vi "CB Discrete LQR.vi"(9 "R":T1, 10 "Q":T1, 11 "State Space Model":T2) -> (1 "X (ricatti solution)":T1, 3 "K (gain matrix)":T1)   [LabVIEW 2020]
uses:
  State-Space/CB State Space.ctl
  <vilib>/Analysis/Matrix/Datatypes/RealMatrix.ctl
  <vilib>/Analysis/7linalg.llb/Real Transpose Matrix.vi
  <vilib>/Analysis/baseanly.llb/Real A x B.vi
  <vilib>/Analysis/Matrix/Numeric/Add/Add - RM,RM.vi
  <vilib>/Analysis/7linalg.llb/Solve Linear Equations (multiple right hand).vi
  <vilib>/Analysis/NI_AALPro.lvlib
  <vilib>/Analysis/NI_AALBase.lvlib
  <vilib>/Analysis/Matrix/NI_Matrix.lvlib
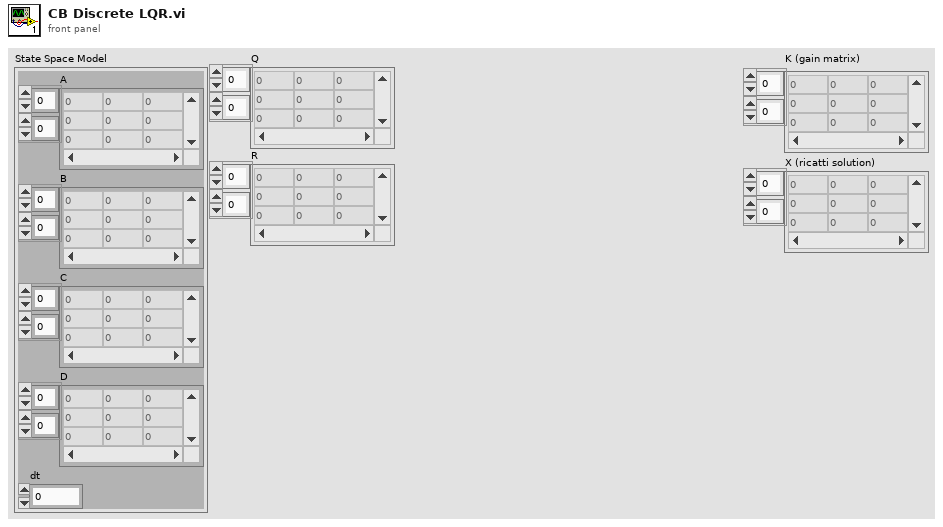
[diagram p1: front panel]
types:
  T1 = typedef "NI_Matrix.lvlib/RealMatrix.ctl" = dbl[][]
  T2 = typedef "CB State Space.ctl" = cluster{"A":T1, "B":T1, "C":T1, "D":T1, "dt":dbl}
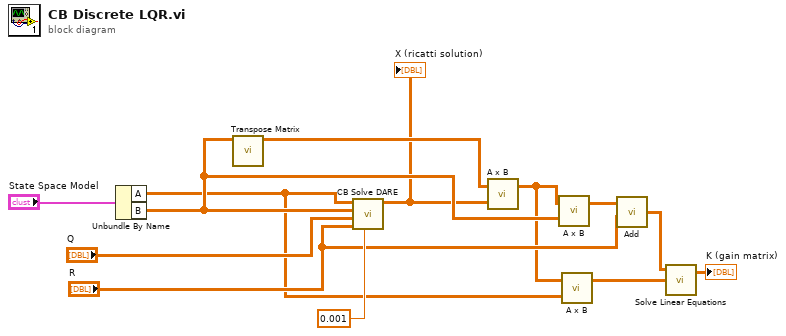
[diagram p0: block diagram]
diagram:
  n1 = Unbundle By Name("State Space Model") -> ("A"=w5:T1, "B"=w9:T1)
  n2 = call-poly <vilib>:"Transpose Matrix.vi"("Input Matrix"=w9) -> ("Matrix Transpose"=w10:T1)  [unwired: 9 in, 1 out]
  n3 = call "CB Solve DARE.vi"("epsilon"=0.001, "R"="R", "Q"="Q", "B"=w9, "A"=w5) -> ("X"=w1:T1)  [unwired: 6 in]
  "X (ricatti solution)" <- w1
  n4 = call-poly <vilib>:"A x B.vi"("B"=w1, "A"=w10) -> ("A x B"=w6:T1)  [unwired: 1 out]
  n5 = call-poly <vilib>:"A x B.vi"("B"=w9, "A"=w6) -> ("A x B"=w8:T1)  [unwired: 1 out]
  n6 = call-poly <vilib>:"A x B.vi"("B"=w5, "A"=w6) -> ("A x B"=w4:T1)  [unwired: 1 out]
  n7 = call-poly <vilib>:"Add.vi"("Real Matrix B"="R", "Real Matrix A"=w8) -> ("A + B"=w3:T1)
  n8 = call-poly <vilib>:"Solve Linear Equations.vi"("Known Matrix"=w4, "Input Matrix"=w3) -> ("Solution Matrix"=→"K (gain matrix)":T1)  [unwired: 1 in, 1 out]
